vi "DAQ Stepper Motor Control (Constant Velocity)_2012.vi"(6 "Clockwise/Counterclockwise?":bool, 7 "Enable Drive":bool, 8 "stop":bool, 9 "Direction Line":tag="Dev3/port1/line4", 10 "Enable Line":tag="Dev3/port1/line1", 11 "Step Pulse Train Frequency (Hz)":dbl=200.0 format="%.6f") -> ()   [LabVIEW 2019]
uses:
  <vilib>/DAQmx/write.llb/DAQmx Write (Digital Bool 1Line 1Point).vi
  <vilib>/DAQmx/create/channels.llb/DAQmx Create Channel (DO-Digital Output).vi
  <vilib>/DAQmx/miscellaneous.llb/DAQmx Fill In Error Info.vi
  <vilib>/DAQmx/create/channels.llb/DAQmx Create Channel (CO-Pulse Generation-Frequency).vi
  <vilib>/DAQmx/configure/timing.llb/DAQmx Timing (Implicit).vi
  <resource>/objmgr/daqmx.rc
panel:
  in  "Step Signal Output Line":tag="/Dev3/PFI2"
  # "The 'Step Signal Output Line', 'Enable Line', and 'Direction Line' each select which digital output channel to use for each control signal."
  # "The motor's actual velocity will be a function\nof the frequency of the pulse train on the step line \nand the drive's steps/revolution setting."
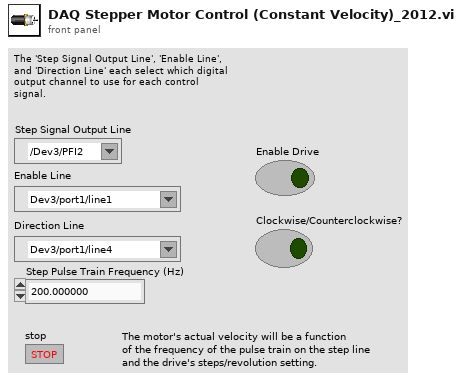
[diagram p1: front panel]
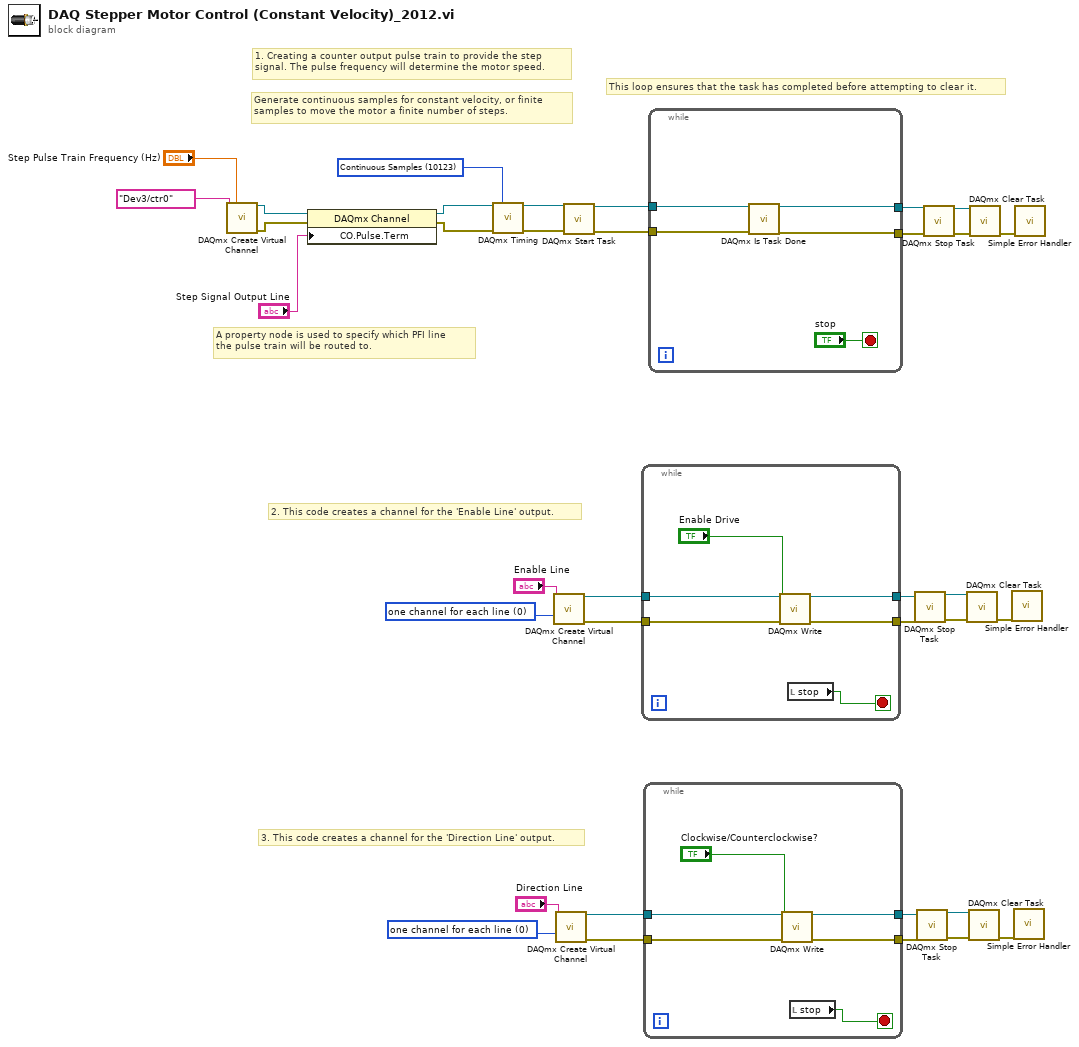
[diagram p0: block diagram]
diagram:
  w3 = 0 items=["one channel for each line", "one channel for all lines"] ("line grouping")
  w18 = 0 items=["one channel for each line", "one channel for all lines"] ("line grouping")
  w34 = 10123 items=["Finite Samples"=10178, "Continuous Samples"=10123, "Hardware Timed Single Point"=12522] ("sample mode")
  # "Generate continuous samples for constant velocity, or finite \nsamples to move the motor a finite number of steps."
  # "A property node is used to specify which PFI line \nthe pulse train will be routed to."
  # "3. This code creates a channel for the 'Direction Line' output."
  # "2. This code creates a channel for the 'Enable Line' output."
  # "This loop ensures that the task has completed before attempting to clear it."
  # "1. Creating a counter output pulse train to provide the step\nsignal. The pulse frequency will determine the motor speed."
  n1 = call-poly <vilib>:"DAQmx Create Virtual Channel.vi"("frequency"="Step Pulse Train Frequency (Hz)", "counter"=tag "Dev3/ctr0") -> ("task out"=w24:refnum<k21>, "error out"=w23:errorcluster)  [unwired: 12 in]
  n2 = property class="DAQmx Channel"(reference=w24, error in=w23, "CO.Pulse.Term"="Step Signal Output Line") -> (reference out=w22:refnum<k21>, error out=w21:errorcluster)
  n3 = call-poly <vilib>:"DAQmx Timing.vi"("task/channels in"=w22, "sample mode"=w34, "error in"=w21) -> ("task out"=w33:refnum<k21>, "error out"=w32:errorcluster)  [unwired: 11 in]
  n4 = call-poly <vilib>:"DAQmx Create Virtual Channel.vi"("lines"="Enable Line", "line grouping"=w18) -> ("task out"=w17:refnum<k21>, "error out"=w16:errorcluster)  [unwired: 12 in]
  n5 = call-poly <vilib>:"DAQmx Create Virtual Channel.vi"("lines"="Direction Line", "line grouping"=w3) -> ("task out"=w4:refnum<k21>, "error out"=w5:errorcluster)  [unwired: 12 in]
  n6 = call <vilib>:"DAQmx Start Task.vi"("task/channels in"=w33, "error in"=w32) -> ("task out"=w31:refnum<k21>, "error out"=w30:errorcluster)  [unwired: 12 in]
  n7 = while {
    tunnel: w17 -> [w40]
    tunnel: w16 -> [w39]
    tunnel: [w38] -> w15
    tunnel: [w37] -> w14
    stop <- w36 stop-if-true
    n8 = call-poly <vilib>:"DAQmx Write.vi"("task/channels in"=w40, "data"="Enable Drive", "error in"=w39) -> ("task out"=w38:refnum<k21>, "error out"=w37:errorcluster)  [unwired: 10 in, 1 out]
    n9 = local read "stop"() -> (w36:bool)
  }
  n10 = while {
    tunnel: w4 -> [w46]
    tunnel: w5 -> [w45]
    tunnel: [w44] -> w6
    tunnel: [w43] -> w7
    stop <- w42 stop-if-true
    n11 = call-poly <vilib>:"DAQmx Write.vi"("task/channels in"=w46, "data"="Clockwise/Counterclockwise?", "error in"=w45) -> ("task out"=w44:refnum<k21>, "error out"=w43:errorcluster)  [unwired: 10 in, 1 out]
    n12 = local read "stop"() -> (w42:bool)
  }
  n13 = while {
    tunnel: w31 -> [w52]
    tunnel: w30 -> [w51]
    tunnel: [w49] -> w29
    tunnel: [w48] -> w28
    stop <- "stop" stop-if-true
    n14 = call <vilib>:"DAQmx Is Task Done.vi"("task/channels in"=w52, "error in"=w51) -> ("task out"=w49:refnum<k21>, "error out"=w48:errorcluster)  [unwired: 11 in, 1 out]
  }
  n15 = call <vilib>:"DAQmx Stop Task.vi"("task/channels in"=w15, "error in"=w14) -> ("task out"=w13:refnum<k21>, "error out"=w12:errorcluster)  [unwired: 12 in]
  n16 = call <vilib>:"DAQmx Stop Task.vi"("task/channels in"=w6, "error in"=w7) -> ("task out"=w8:refnum<k21>, "error out"=w9:errorcluster)  [unwired: 12 in]
  n17 = call <vilib>:"DAQmx Stop Task.vi"("task/channels in"=w29, "error in"=w28) -> ("task out"=w27:refnum<k21>, "error out"=w26:errorcluster)  [unwired: 12 in]
  n18 = call <vilib>:"DAQmx Clear Task.vi"("task in"=w13, "error in"=w12) -> ("error out"=w11:errorcluster)  [unwired: 13 in]
  n19 = call <vilib>:"DAQmx Clear Task.vi"("task in"=w8, "error in"=w9) -> ("error out"=w10:errorcluster)  [unwired: 13 in]
  n20 = call <vilib>:"DAQmx Clear Task.vi"("task in"=w27, "error in"=w26) -> ("error out"=w25:errorcluster)  [unwired: 13 in]
  n21 = call <vilib>:"Simple Error Handler.vi"("error in (no error)"=w11) -> ()  [unwired: 4 in, 5 out]
  n22 = call <vilib>:"Simple Error Handler.vi"("error in (no error)"=w10) -> ()  [unwired: 4 in, 5 out]
  n23 = call <vilib>:"Simple Error Handler.vi"("error in (no error)"=w25) -> ()  [unwired: 4 in, 5 out]
